vi "AlliGator Decay Fit Parameter Map Context Menu Handler.vi"(8 "Error In":errorcluster, 11 "Image Event Data":T1) -> (0 "Error Out":errorcluster, 3 "AlliGator Actions":T4[](array[typedef]))   [LabVIEW 2021, in "AlliGator Decay Fit Parameter Map.lvlib"]
doc: "Decay Fit Parameter Map contextual menu handler."
uses:
  AlliGator Decay Fit Parameter Map.lvlib
  AlliGator Q Element.ctl
  AlliGator Q Event.ctl
  Image/Image Display Event.ctl
  Image/Image Control Refnum.ctl
  <vilib>/Utility/miscctls.llb/LVPoint32TypeDef.ctl
  Image/Image Display to Clipboard Options.ctl
  AlliGator Variables List.ctl
  Files/Load-Save File Info.ctl
  Variant/Variant to Data/Variant to I32.vi
  AlliGator Action Engine.lvlib
  Image/Image.lvlib
  Files/Files.lvlib
  AlliGator Globals, Variables & Constants.lvlib
  Variant/Variant to Data/Variant to Data.lvlib
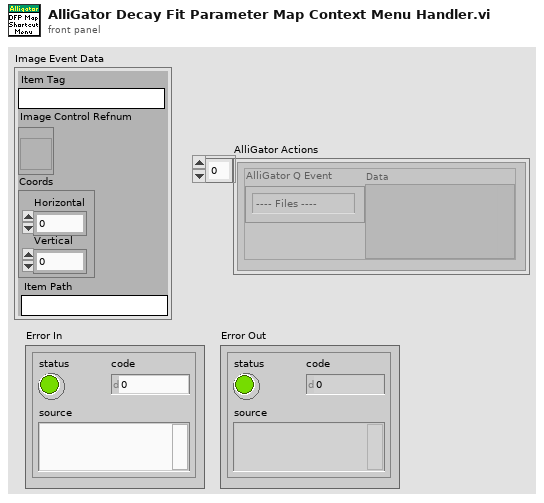
[diagram p1: front panel]
types:
  T1 = typedef "Image.lvlib/Image Display Event.ctl" = cluster{"Item Tag":string, "Image Control Refnum":T2, "Coords":T3, "Item Path":string}
  T2 = typedef "Image.lvlib/Image Control Refnum.ctl" = refnum<vi>
  T3 = typedef "LVPoint32TypeDef.ctl" = cluster{"Horizontal":i32, "Vertical":i32}
  T4 = typedef "AlliGator Action Engine.lvlib/AlliGator Q Element.ctl" = cluster{"AlliGator Q Event":T5, "Data":variant}
  T5 = typedef "AlliGator Action Engine.lvlib/AlliGator Q Event.ctl" = enum16{"---- Files ----", "Files:Set Batch Export Files To Save", "Files:Set Dataset Loading & Pre-processing Options", "Files:Check #Frames in Dataset", "Files:Increment Frame Index", "Files:Open Mask Image", "Files:Open White Light Image", "Files:Open Single Dataset", "Files:New Folder of Folders Selected", "Files:Load File (all Types)_Scriptable", "Files:Move Flattened Series to Folders Series", "Files:Select Folder", "Files:Load FLI Dataset", "Files:Load Swiss SPAD 1 Dataset", "Files:Load Swiss SPAD 2 Dataset", "Files:Load .sdt FLI Dataset", "Files:Load .ptu FLI Dataset", "Files:Load .bin FLI Dataset", "Files:Load Single Gate Image Folder", "Files:Load I/m/phi Dataset (deprecated)", "Files:Load Single Image", "Files:Subtract Background File", "Files:Export FLI Dataset", "Files:Load HDF5 FLI Dataset", "Files:Set Destination File Path", "Files:Save Mask Image", "Files:Batch Conversion", "Files:New Folder Selected", "Files:Close FLI Dataset", "Files:Close FLI Dataset Series", "Files:Close White Light Image", "Files:Close Mask Image", "---- FLI Dataset ----", "FLI Dataset:Channel Arithmetic", "FLI Dataset:Export Average Lifetime Map as ASCII", "FLI Dataset:Export User-Defined Quantity Map as ASCII", "FLI Dataset:Python Function FLI Dataset Event", "FLI Dataset:ROI Analysis", "FLI Dataset:Tilted Logistic Square Gated IRF Characteristics Map", "FLI Dataset:Logistic Square Gated IRF Characteristics Map", "FLI Dataset:Square Gated IRF Characteristics Map", "FLI Dataset:Multi-ROI Single-Pixel Phasor Analysis", "FLI Dataset:Multi-ROI Single-Pixel NLSF Analysis", "FLI Dataset:All ROIs IRF Extraction", "FLI Dataset:All ROIs Decay Fit Non-Interactive (Fast + Individual IRF)", "FLI Dataset:All ROIs Phasor Analysis", "FLI Dataset:All ROIs Decay Fit", "FLI Dataset:Fluorescence Decay Statistics", "FLI Dataset:Update Decay Statistics Graph", "FLI Dataset:Get Decay from ROI", "FLI Dataset:All ROIs Average Lifetimes", "---- FLI Dataset Series ----", "FLI Dataset Series:Sum All Datasets in Series", "FLI Dataset Series:Add Dataset to Accumulated Dataset", "FLI Dataset Series:Display Accumulated Dataset", "FLI Dataset Series:Clear Dataset Series Sum", "FLI Dataset Series:Time-Series Analysis (NLSF)", "FLI Dataset Series:Time-Series Analysis (Phasor)", "---- Image ----", "Image:Update Image Profile Plots", "Image:Image Histogram Cursor Move", "Image:Image Histogram", "Image:Image Contrast", "Image:Set Image Histogram Cursor Move Flag", "Image:Clear Image Overlay", "Image:Use ROI as Search Area", "Image:Set ROI Diameter", "Image:Save Image Data as TIFF", "Image:Save Displayed Image with Overlay", "Image:Save Image Overlay Only", "Image:Save Image as Hot Pixel Mask", "Image:Change Source Image Color Palette", "Image:Copy Image to Clipboard", "Image:Source Image ROI Selection", "Image:Delete All ROIs", "Image:Delete All Unselected ROIs", "Image:Delete ROI", "Image:Merge All ROIs", "Image:Store ROI", "Image:Source Image ROI Storage", "Image:Export ROI Description to Notebook", "Image:Save ROI", "Image:Load ROI", "Image:Paste ROI Definition", "Image:Clear ROI", "Image:Identify ROIs in Mask Image", "Image:Create Complementary ROI", "Image:Create Contour ROI", "Image:Create ROI(s) from Pixels with Peak above Min_Scriptable", "Image:Create ROI(s) from Pixels with Intensity above Min_Scriptable", "Image:Compute ROI Statistics", "Image:Delete ROI(s) based on ROI Characteristics", "Image:Create ROI Grid", "Image:ROI to Individual Pixel ROIs", "Image:Python Function Source Image Event", "Image:Show Phasor Calibration Map ROI Centers", "Image:Convert ROI to Mask Image", "Image:Mouse Move", "Image:Mouse Up", "Image:Set Source Image Mouse Move Flag", "Image:Add Scale Bar Overlay", "Image:Delete Existing ROIs Option", "---- Decay ----", "Decay:Clear IRF/Reference Plot", "Decay:Clear Local IRFs", "Decay:Add Decay to Graph", "Decay:Smoothen Plot", "Decay:Smoothen Plot Tail", "Decay:Average Selected Plots", "Decay:Extract IRF", "Decay:Optimal IRF Extraction", "Decay:Threshold IRF", "Decay:Fit to Model IRF", "Decay:Fit IRF to Square Gate", "Decay:Fit IRF to Logistic Square Gate", "Decay:Fit IRF to Tilted Logistic Square Gate", "Decay:Create Bounding Cursors Set", "Decay:Export Bounding Cursors Definition to Notebook", "Decay:Denoise Plot", "Decay:Compute Cumulative Function", "Decay:Use as Reference Decay", "Decay:Show Reference Decay/IRF", "Decay:Extrapolate Decay", "Decay:Create Head & Tail Bounding Cursors", "Decay:Store Cursor-defined Head & Tail Fractions", "Decay:Rebin Plot", "Decay:1-Normalize Decay", "Decay:[0-1]-Normalize Plot", "Decay:Straighten Decay", "Decay:Shift Decay", "Decay:Fold Decay", "Decay:Fit Decay", "Decay:Global Fit of Selected Decays", "Decay:Post Global Fit Script", "Decay:Add Global Fit Parameters to Graph", "Decay:Add Decay Parameter(s) to Plot (Graph)", "Decay:Export Decay to Phasor Graph", "Decay:Plot Decay Shifts", "Decay:Compute Average Lifetime", "Decay:Plot Convolution", "Decay:Graph Tip Strip Update", "---- Decay Statistics ----", "Decay Statistics:Tip Strip Update", "---- Intensity Time Trace ----", "Intensity Time Trace:Use File Timestamp", "Intensity Time Trace:Load Intensity Corrections File", "Intensity Time Trace:Clear Intensity Corrections File", "Intensity Time Trace:Tip Strip Update", "---- Phasor Plot ----", "Phasor Plot:Build Phasor Plot", "Phasor Plot:Change Phasor Plot Color Palette", "Phasor Plot:Adjust Phasor Plot Display Range", "Phasor Plot:Highlight Image ROI in Phasor Plot", "Phasor Plot:Save Phasor Plot Image with Overlay", "Phasor Plot:Export Complex Phasor Map", "Phasor Plot:Export Phasor Ratio Map", "Phasor Plot:Export Average Lifetime Map", "Phasor Plot:Compute Phase Lifetime Histogram", "Phasor Plot:Compute Phasor Ratio Histogram", "Phasor Plot:Compute Phase Lifetime vs Intensity Scatter Plot", "Phasor Plot:Weber 2-Component Decomposition", "Phasor Plot:Update Phasor Color Map Vertices", "Phasor Plot:Clear Phasor Overlay", "Phasor Plot:Use Segment Extremities as References", "Phasor Plot:Use UC/Segment Intersections as References", "Phasor Plot:Use UC/Principal Axis Intersections as References", "Phasor Plot:Use UC/Linear Fit Intersections as References", "Phasor Plot:Update Phasor Plot Reference", "Phasor Plot:Show Local Phasor Info in Phasor Plot", "Phasor Plot:Update Phasor Plot State", "Phasor Plot:Phasor Plot ROI Storage", "Phasor Plot:Phasor Plot ROI Selection", "Phasor Plot:Python Function Phasor Plot Event", "Phasor Plot:Overlay Phasor ROI, Ratio or Map in Source Image", "Phasor Plot:Compute Decay of Selected Phasors", "Phasor Plot:Phasor at Image Pixel", "Phasor Plot:Mouse Move", "Phasor Plot:Mouse Up", "Phasor Plot:Display Range Mouse Move", "Phasor Plot:Set Mouse Move Flag", "---- Phasor Graph ----", "Phasor Graph:Calibrated Phasor Map Series", "Phasor Graph:Whole Image Phasor Scatter Plot (Todo)", "Phasor Graph:Get Phasor Value", "Phasor Graph:Create New Phasor Plot Dialog", "Phasor Graph:Update Last Phasor Value", "Phasor Graph:Update Phasor (m, phi)", "Phasor Graph:Remove Single Phasor from Plot", "Phasor Graph:Add Single Phasor to Plot", "Phasor Graph:Remove Phasor Plot", "Phasor Graph:Remove Selected Phasor Plots", "Phasor Graph:Clear Phasor Data", "Phasor Graph:Clear Phasor Graph", "Phasor Graph:Cursor Move", "Phasor Graph:Draw Cursor Connecting Line", "Phasor Graph:Clear Cursor Connecting Line", "Phasor Graph:Find UC Intersection", "Phasor Graph:Use UC/Cursor-Defined Line Intersections", "Phasor Graph:Use Selected Plots Fitted Line/UC Intersections", "Phasor Graph:Use Selected Plots Principal Axis/UC Intersections", "Phasor Graph:Show Single Phasor", "Phasor Graph:Save Single Phasor Plot", "Phasor Graph:Save All Phasor Plots", "Phasor Graph:Load Phasor Plot(s)", "Phasor Graph:Phasor Multiplication", "Phasor Graph:Compute Average Phasor", "Phasor Graph:Compute Multiple Average Phasors (Selected Plots)", "Phasor Graph:Export Single Phasor Plot Phase Lifetimes", "Phasor Graph:Phase Lifetime Trajectory", "Phasor Graph:Phase Lifetime vs Intensity Scatter Plot (deprecated)", "Phasor Graph:Parameter 2 vs Parameter 1 Scatter Plot", "Phasor Graph:Use Cursor n Location", "Phasor Graph:Set Reference n to Current Phase Lifetime Value", "Phasor Graph:Set Reference n to Lifetime Value", "Phasor Graph:Set Cursor n Location", "Phasor Graph:Save Phasor Graph Image", "Phasor Graph:Update SEPL Plot", "Phasor Graph:Export Single Phasor Plot Data", "Phasor Graph:Export Selected Phasor Plots Data", "Phasor Graph:Python Function Phasor Graph Event", "Phasor Graph:Tip Strip Update", "---- Calibration ----", "Calibration:Set Calibration Type", "Calibration:Load/Save Phasor Calibration", "Calibration:Load/Save Phasor Calibration Series", "Calibration:Load/Save Phasor Calibration Map", "Calibration:Use as Calibration", "Calibration:Compute Optimal Calibration from Phasor References", "Calibration:Clear Phasor Calibration", "Calibration:Single Phasor Calibration Information", "Calibration:Use as Calibration Series", "Calibration:Use as Calibration Map", "Calibration:Clear Calibration Series", "Calibration:Phasor Calibration Series Information", "Calibration:Clear Calibration Map", "Calibration:Phasor Calibration Map Information", "Calibration:Apply Phasor Calibration", "Calibration:Update Single Plot Calibration", "Calibration:Update Multiple Plots Calibration", "Calibration:Clear Single Plot Calibration", "Calibration:Clear All Plots Calibrations", "Calibration:Clear Plot(s) Calibration(s)?", "Calibration:Phasor Calibration Maps (# Gates Series)", "---- Phasor Ratio ----", "Phasor Ratio:Clear Reference n", "Phasor Ratio:Toggle Selected Plot(s)  Lock to Reference 1", "Phasor Ratio:Use as Reference n", "Phasor Ratio:Send Reference n to Notebook", "Phasor Ratio:Toggle Selected Plot(s)  Lock to Reference 2", "Phasor Ratio:Compute Phasor Ratio at Mouse Location", "Phasor Ratio:Compute Phasor Plot's Average Phasor Ratio", "Phasor Ratio:Compute Time-Series Phasor Ratios", "Phasor Ratio:Fit Line to Phasor Ratio Plot", "Phasor Ratio:Save References", "Phasor Ratio:Load References", "Phasor Ratio:Update Phasor Reference 1", "Phasor Ratio:Update Phasor Reference 2", "Phasor Ratio:Move Cursor n to Reference n", "Phasor Ratio:Use as Phasor Reference 1 Lifetime", "Phasor Ratio:Use as Phasor Reference 2 Lifetime", "Phasor Ratio:Export Phasor Ratio Map as ASCII", "Phasor Ratio:Tip Strip Update", "---- Lifetime & Other Parameters Graph ----", "Lifetime:Tip Strip Update", "---- Decay Fit Parameter Map ----", "Decay Fit Parameter Map:Export ROI NLSF Data as ASCII", "Decay Fit Parameter Map:Set Decay Fit  Parameter Map Selection", "Decay Fit Parameter Map:Build Decay Fit Parameter Map", "Decay Fit Parameter Map:Change Decay Fit Parameter Map Color Palette", "Decay Fit Parameter Map:Export Decay Fit Parameter Map Data as ASCII", "Decay Fit Parameter Map:Export All Decay Fit Parameter Maps Data as ASCII", "Decay Fit Parameter Map:Send Map Data to Lifetime Graph", "Decay Fit Parameter Map:Save Decay Fit Parameter Map Image", "Decay Fit Parameter Map:Save-Load IRFs & Fit Data", "Decay Fit Parameter Map:Update Local Decay Plots", "Decay Fit Parameter Map:Python Function Decay Fit Parameters Map Event", "Decay Fit Parameter Map:Overlay Decay Fit Parameter Map in Source Image", "Decay Fit Parameter Map:Plot Map Data vs Intensity", "Decay Fit Parameter Map:Mouse Up", "Decay Fit Parameter Map:Display Range Mouse Move", "---- Generic Graph ----", "Generic Graph:Generic XY Graph Event", "Generic Graph:Python Function XY Graph Event", "Generic Graph:New Plot", "Generic Graph:Save Plot", "Generic Graph:XY Plot Histogram", "Generic Graph:Set XY Graph Plot Name", "Generic Graph:Set Last Cursor Style", "Generic Graph:Tip Strip Update", "---- GUI ----", "GUI:Start Script", "GUI:Type of Displayed Image Changed", "GUI:Gate Image Slide Changed", "GUI:Show Busy Icon", "GUI:Show Busy Icon & Abort Button", "GUI:Hide Busy Icon", "GUI:Hide Busy Icon & Abort Button", "GUI:Abort", "GUI:End Script", "GUI:Start Timing", "GUI:End Timing", "GUI:Set State Indicator", "GUI:Send Parameters JSON Strings to Clipboard", "GUI:Set Gate Step", "GUI:Idle", "GUI:Initialization", "GUI:Quit", "GUI:Increment Dataset Index", "GUI:Set Dataset Index to -1", "GUI:Time Series Slider Moved", "GUI:Time Series Slider Changed", "GUI:Toggle Playback or Loop", "GUI:Playback Script", "GUI:Set Phasor Frequency", "GUI:Open Window", "GUI:Start Test Script", "GUI:End Test Script", "DEBUG"}
  T6 = typedef "Image.lvlib/Image Display to Clipboard Options.ctl" = cluster{"Include Overlay (T)":bool, "Image Only (T)":bool}
  T7 = typedef "AlliGator Globals, Variables & Constants.lvlib/AlliGator Variables List.ctl" = enum16{"---- GUI ----", "Initialization Status", "State Indicators Refnum", "Original AlliGator Menu Items", "Current Action Loop State", "Script in progress", "Playback", "Loop Playback", "Search ROI Used", "Search ROI", "Decay Graph Max Legend Size", "Intensity Graph Max Legend Size", "Decay Statistics Graph Max Legend Size", "Phasor Graph Max Legend Size", "Phasor Ratio Graph Max Legend Size", "Lifetime Graph Max Legend Size", "---- Files ----", "Export Dataset Frames as Individual Files", "Show Batch Export Help Balloons", "Frames in Dataset", "ptu File Frame Start Indices", "Current Frame in Dataset", "Current Frame Timestamp", "------ Python Plugins ------", "Python Plugins Information", "Python Session", "Valid Python Session?", "---- Source Image ----", "Dataset Loaded", "Dataset Metadata", "Dataset Channel", "Dataset Data Description", "Background Dataset Metadata", "Background Dataset Channel", "Background Dataset Data Description", "Background File Subtraction", "Background File Path", "Background File Pile-up Correction", "Background File Pixel Well Capacity", "Background File Scaling Factor", "Source Image ROIs", "Current Source Image ROI", "Source Image ROI Event Refnum", "X_Source Image Display Range", "X_Source Image Palette Information", "Source Image Palette List", "Source Image Scale", "Current Dataset Load Settings", "Source Image:ROI Overlay Color", "---- Image Profile Window ----", "Image Profile:Overlay ROI in Source Image", "Image Profile Window Event Refnum", "Image Profile:IntensityType", "Image Profile:Intensity Average Type", "Image Profile:Intensity-weighted SDV", "Image Profile:Box Profile Type", "Image Profile Window Open", "Image Profile:Plotted Fit Parameter", "X_Type of Displayed Image", "X_Time Gate Slider", "Dataset Path", "Source Image Overlay to Erase", "Is Displayed Image Accumulated", "White Light Image Modified", "Mask Image Modified", "Macrotime Gate Separation", "------ Phasor Graph -------", "Phasor Graph:Show Line", "---- Phasor Plot ---", "Phasor Plot Parameters Changed", "FLI Dataset Modified since last Phasor Plot Calculation", "Phasor Harmonics Data", "Selected Phasor Harmonics", "Phasor Harmonic Manager Event Refnum", "Phasor Plot ROIs", "Current Phasor Plot ROI", "Phasor Plot ROI Event Refnum", "Phasor Plot Image Reference Points", "Phasor Plot Computed", "Phasor Plot Palette Information", "Phasor Plot Palette List", "Phasor Ratio Palette Information", "Phasor Ratio Palette List", "Phasor Image Scale", "Phasor Plot Image Overlay to Erase", "Phasor Plot Image Elements to Update", "Current Phasor Plot Calculation Parameters", "Current Phasor Calibration Options", "Reset Cumulated Phasor Plot", "Phasor Ratio Reference 1", "Phasor Ratio Lifetime Reference 1", "Phasor Ratio Reference 1 Frequency", "Phasor Ratio Reference 2", "Phasor Ratio Lifetime Reference 2", "Phasor Ratio Reference 2 Frequency", "---- Decay Analysis ----", "Number of Selected Decays to Fit", "LS Fit Results", "LAR Fit Results", "BS Fit Results", "Last Decay Max - Min", "Best Fit Parameters", "Best Fit Parameter Names", "Actual Size X", "Actual Size Y", "Binning X", "Binning Y", "Actual # Gates", "Dataset Number", "Gates to...", "Gates Skipped", "Gates to keep", "Gate Step", "Gate Separation", "Reversed Gates", "Pile-up Correction", "Pixel Well Capacity", "Background Subtracted", "Background Subtraction Method", "Background Definition Range", "Background File (deprecated)", "Number of Dataset Accumulated", "Array of Accumulated Dataset Paths", "Do Averaged Datasets", "Destination File Path", "Process Plot Target", "Use 1/D as Phasor Frequency", "---- Decay Fit Parameter Map -----", "Decay Fit Parameter Map Palette Information", "Decay Fit Parameter Map Palette List", "Local Decay Graph Window Event Refnum", "------- Local Decay Window ---------", "Use normalized IRF for convolution", "----- Miscellaneous ----", "Skippable Dialog Windows Status"}
  T8 = typedef "Files.lvlib/Load-Save File Info.ctl" = cluster{"Load/Save":bool, "File Path":path}
  T9 = cluster{"Image Control Refnum":T2, "Image to Clipboard Options":T6}
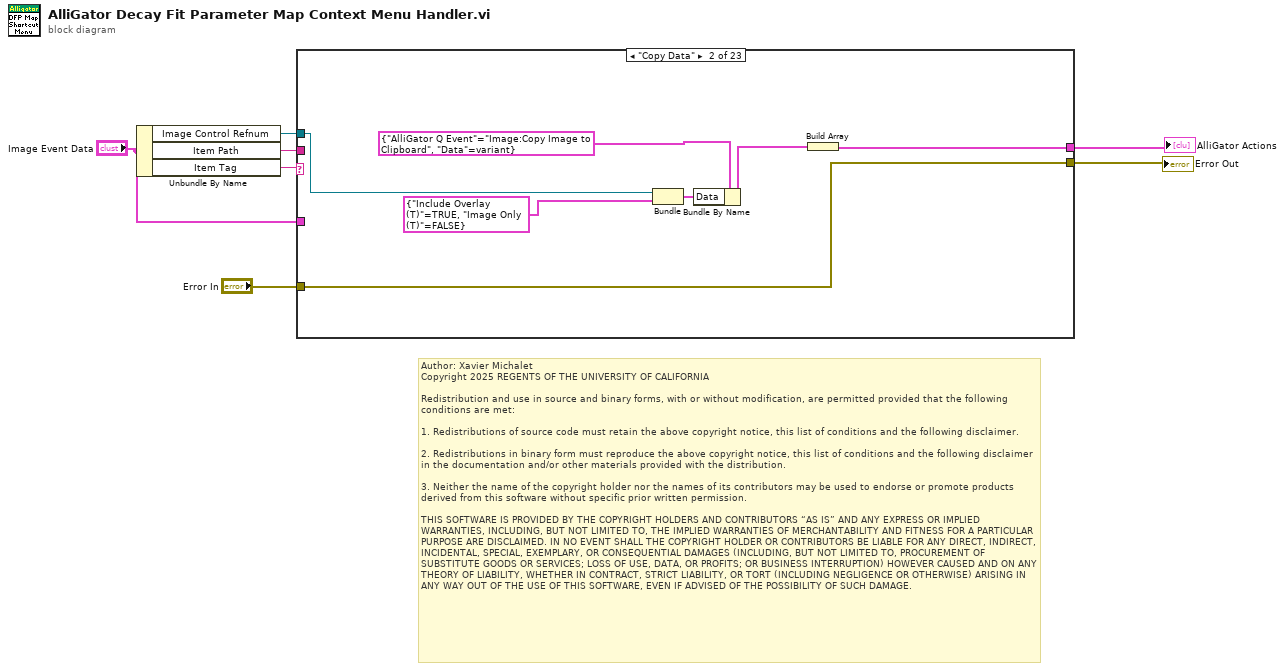
[diagram p0: block diagram]
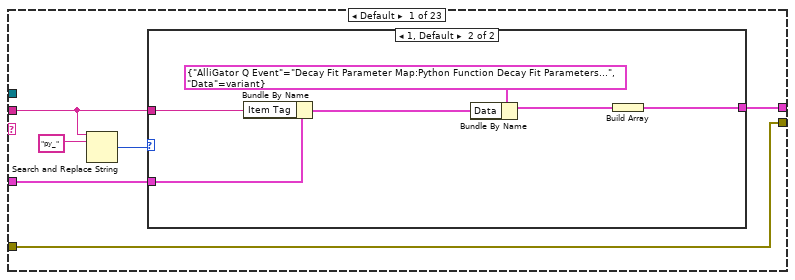
[diagram p2: hidden frame]
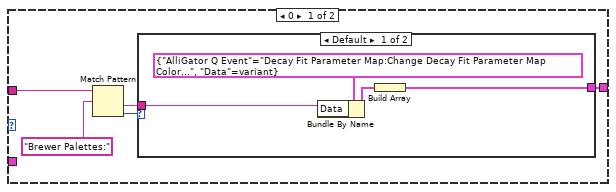
[diagram p3: hidden frame]
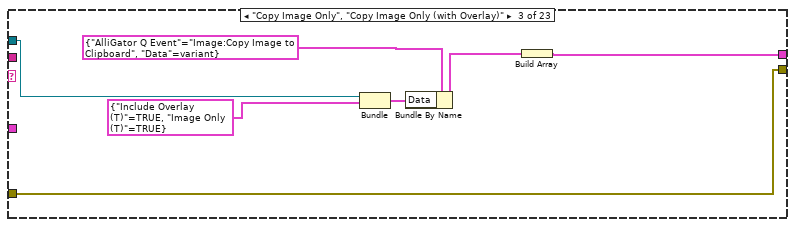
[diagram p5: hidden frame]
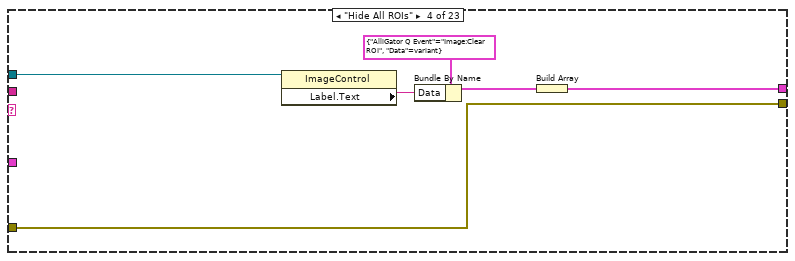
[diagram p6: hidden frame]
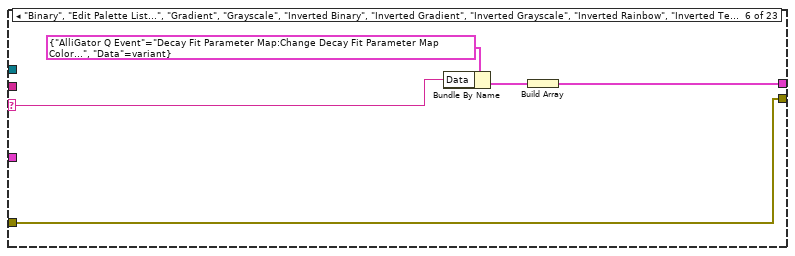
[diagram p8: hidden frame]
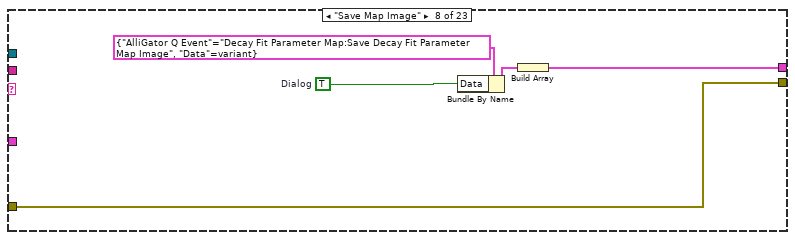
[diagram p10: hidden frame]
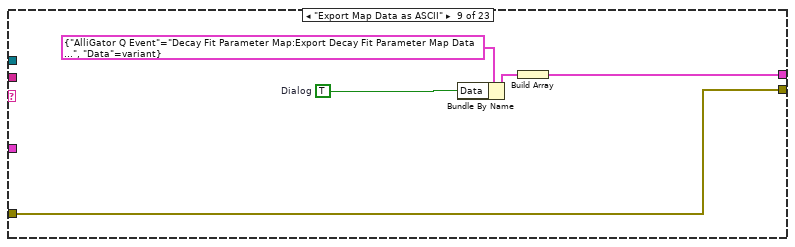
[diagram p11: hidden frame]
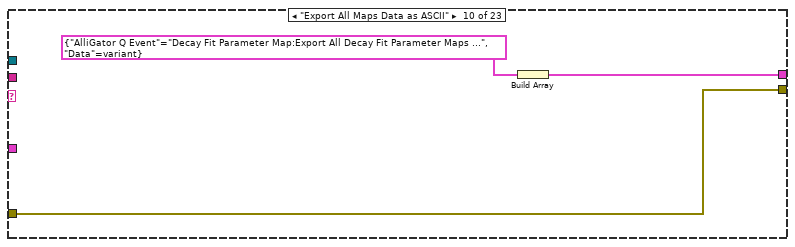
[diagram p12: hidden frame]
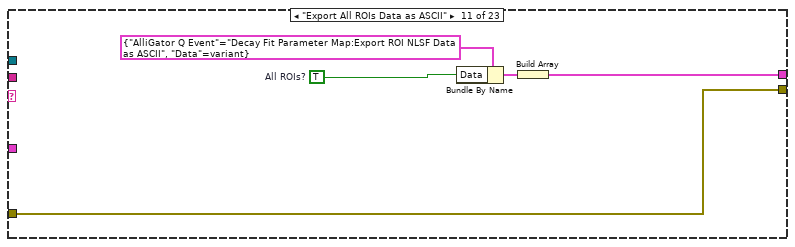
[diagram p13: hidden frame]
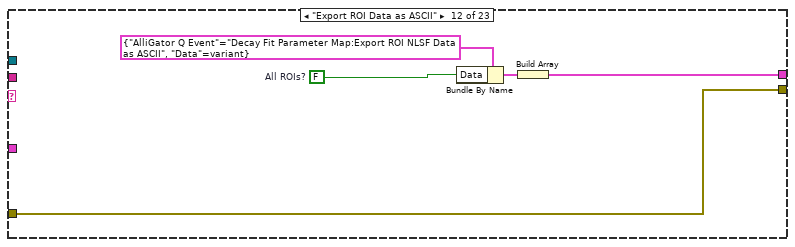
[diagram p14: hidden frame]
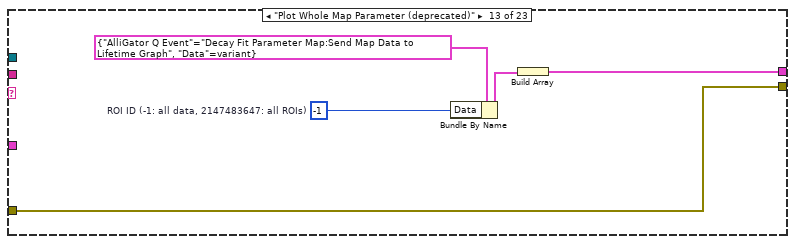
[diagram p15: hidden frame]
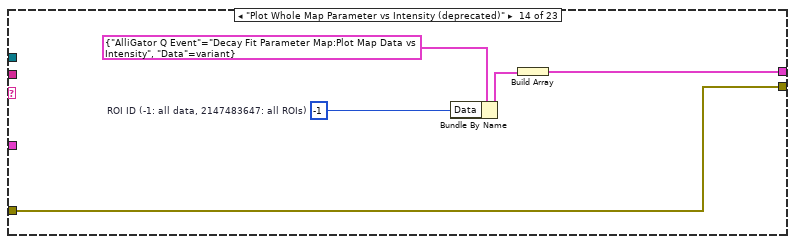
[diagram p16: hidden frame]
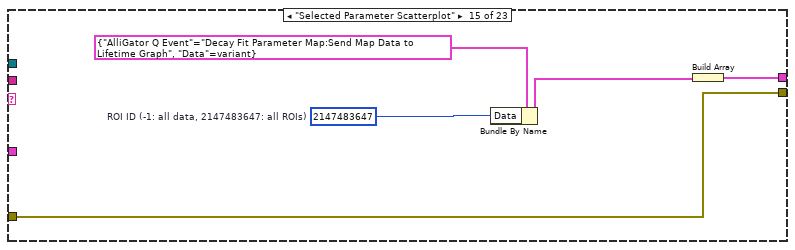
[diagram p17: hidden frame]
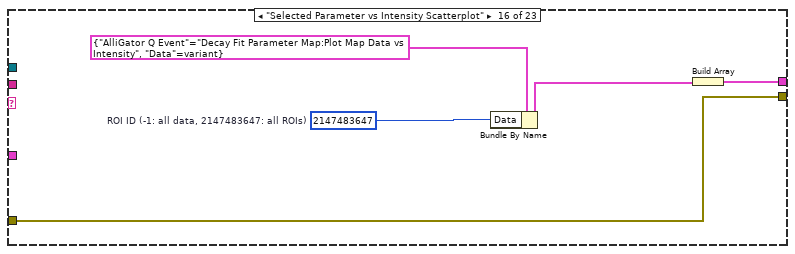
[diagram p18: hidden frame]
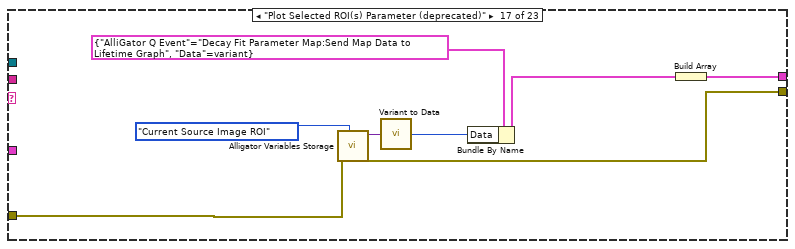
[diagram p19: hidden frame]
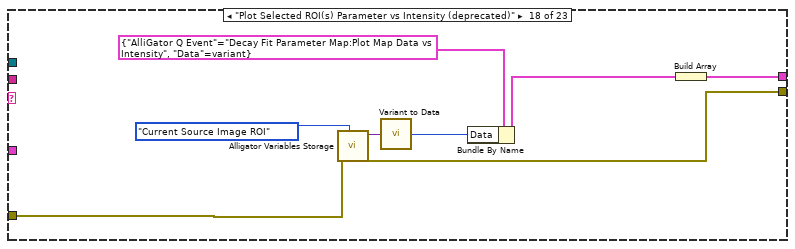
[diagram p20: hidden frame]
diagram:
  # "Author: Xavier Michalet\nCopyright 2025 REGENTS OF THE UNIVERSITY OF CALIFORNIA\n\nRedistribution and use in source and binary forms, with or without modification, are permitted provided that the following conditions are met:\n\n1. Redistributions of source code must retain the above copyright notice, this list of conditions and the following disclaimer.\n\n2. Redistributions in binary form must reproduce the above copyright notice, this list of conditions and the following disclaimer in the documentation and/or other materials provided with the distribution.\n\n3. Neither the name of the copyright holder nor the names of its contributors may be used to endorse or promote products derived from this software without specific prior written permission.\n\nTHIS SOFTWARE IS PROVIDED BY THE COPYRIGHT HOLDERS AND CONTRIBUTORS “AS IS” AND ANY EXPRESS OR IMPLIED WARRANTIES, INCLUDING, BUT NOT LIMITED TO, THE IMPLIED WARRANTIES OF MERCHANTABILITY AND FITNESS FOR A PARTICULAR PURPOSE ARE DISCLAIMED. IN NO EVENT SHALL THE COPYRIGHT HOLDER OR CONTRIBUTORS BE LIABLE FOR ANY DIRECT, INDIRECT, INCIDENTAL, SPECIAL, EXEMPLARY, OR CONSEQUENTIAL DAMAGES (INCLUDING, BUT NOT LIMITED TO, PROCUREMENT OF SUBSTITUTE GOODS OR SERVICES; LOSS OF USE, DATA, OR PROFITS; OR BUSINESS INTERRUPTION) HOWEVER CAUSED AND ON ANY THEORY OF LIABILITY, WHETHER IN CONTRACT, STRICT LIABILITY, OR TORT (INCLUDING NEGLIGENCE OR OTHERWISE) ARISING IN ANY WAY OUT OF THE USE OF THIS SOFTWARE, EVEN IF ADVISED OF THE POSSIBILITY OF SUCH DAMAGE."
  n1 = Unbundle By Name("Image Event Data") -> ("Image Control Refnum"=w4:T2, "Item Path"=w3:string, "Item Tag"=w2:string)
  n2 = case shown="\"Copy Data\"" w2 {
    selector: w2 -> [_ _ _ _ _ w52 _ _ _ _ _ _ _ _ _ _ _ _ _ _ _ _ _]
    tunnel: w4 -> [_ w31 w38 w43 _ _ _ _ _ _ _ _ _ _ _ _ _ _ _ _ _ w132 w134]
    tunnel: w3 -> [w8 _ _ _ _ _ _ _ _ _ _ _ _ _ _ _ _ _ _ _ _ _ _]
    tunnel: [w13 w30 w37 w44 _ w51 _ w57 w62 w67 w72 w77 w82 w87 w92 w97 w106 w114 w120 w127 _ _ _] -> w7
    tunnel: "Error In" -> [w12 w29 w36 w48 w49 w50 w55 w60 w65 w68 w73 w78 w83 w88 w93 w98 w102 w110 w121 w128 w129 w130 w133]
    tunnel: [w12 w29 w36 w48 w49 w50 w55 w60 w65 w68 w73 w78 w83 w88 w93 w98 w101 w109 w121 w128 w129 w130 w133] -> w5
    tunnel: "Image Event Data" -> [w9 _ _ _ _ _ _ _ _ _ _ _ _ _ _ _ _ _ _ _ _ _ _]
    frame Default {
      n3 = Search and Replace String(input string=w8, search string="py_") -> (number of replacements=w10:i32)  [unwired: 6 in, 3 out]
      n4 = case shown="1, Default" w10 {
        tunnel: [w15 w23] -> w13
        tunnel: w8 -> [w14 w26]
        tunnel: w9 -> [_ w24]
        frame 0 {
          n5 = Match Pattern(string=w14, regular expression="Brewer Palettes:") -> (after substring=w16:string, offset past match=w17:i32)  [unwired: 1 in, 2 out]
          n6 = case shown="Default" w17 {
            tunnel: w16 -> [w20 _]
            tunnel: [w19 _] -> w15
            frame Default {
              n7 = Bundle By Name(cluster=T4 {"AlliGator Q Event"=enum."Decay Fit Parameter Map:Change Decay Fit Parameter Map Color Palette", "Data"=variant} ("element"), "Data"=w20) -> (w21:T4)
              n8 = Build Array(w21) -> (w19:T4[])
            }
            frame -1 {
            }
          }
        }
        frame 1, Default {
          n9 = Bundle By Name(cluster=w24, "Item Tag"=w26) -> (w27:T1)
          n10 = Bundle By Name(cluster=T4 {"AlliGator Q Event"=enum."Decay Fit Parameter Map:Python Function Decay Fit Parameters Map Event", "Data"=variant}, "Data"=w27) -> (w25:T4)
          n11 = Build Array(w25) -> (w23:T4[])
        }
      }
    }
    frame "Copy Data" {
      n12 = Bundle("Image Control Refnum"=w31, "Image to Clipboard Options"=T6 {"Include Overlay (T)"=TRUE, "Image Only (T)"=FALSE}) -> (w32:T9)  [unwired: 1 in]
      n13 = Bundle By Name(cluster=T4 {"AlliGator Q Event"=enum."Image:Copy Image to Clipboard", "Data"=variant} ("element"), "Data"=w32) -> (w34:T4)
      n14 = Build Array(w34) -> (w30:T4[])
    }
    frame "Copy Image Only", "Copy Image Only (with Overlay)" {
      n15 = Bundle("Image Control Refnum"=w38, "Image to Clipboard Options"=T6 {"Include Overlay (T)"=TRUE, "Image Only (T)"=TRUE}) -> (w39:T9)  [unwired: 1 in]
      n16 = Bundle By Name(cluster=T4 {"AlliGator Q Event"=enum."Image:Copy Image to Clipboard", "Data"=variant} ("element"), "Data"=w39) -> (w41:T4)
      n17 = Build Array(w41) -> (w37:T4[])
    }
    frame "Hide All ROIs" {
      n18 = property class="ImageControl"(reference=w43) -> ("Label.Text"=w45:string)  [unwired: 1 in, 2 out]
      n19 = Bundle By Name(cluster=T4 {"AlliGator Q Event"=enum."Image:Clear ROI", "Data"=variant} ("element"), "Data"=w45) -> (w46:T4)
      n20 = Build Array(w46) -> (w44:T4[])
    }
    frame "---------Palette----------" {
    }
    frame "Binary", "Edit Palette List...", "Gradient", "Grayscale", "Inverted Binary", "Inverted Gradient", "Inverted Grayscale", "Inverted Rainbow", "Inverted Temperature", "Rainbow", "Select New Palette...", "Temperature" {
      n21 = Bundle By Name(cluster=T4 {"AlliGator Q Event"=enum."Decay Fit Parameter Map:Change Decay Fit Parameter Map Color Palette", "Data"=variant} ("element"), "Data"=w52) -> (w53:T4)
      n22 = Build Array(w53) -> (w51:T4[])
    }
    frame "--------- Others  ---------" {
    }
    frame "Save Map Image" {
      w56 = TRUE  # Dialog
      n23 = Bundle By Name(cluster=T4 {"AlliGator Q Event"=enum."Decay Fit Parameter Map:Save Decay Fit Parameter Map Image", "Data"=variant} ("Time-Gated Phasor Q Element"), "Data"=w56) -> (w58:T4)
      n24 = Build Array(w58) -> (w57:T4[])
    }
    frame "Export Map Data as ASCII" {
      w61 = TRUE  # Dialog
      n25 = Bundle By Name(cluster=T4 {"AlliGator Q Event"=enum."Decay Fit Parameter Map:Export Decay Fit Parameter Map Data as ASCII", "Data"=variant} ("Time-Gated Phasor Q Element"), "Data"=w61) -> (w63:T4)
      n26 = Build Array(w63) -> (w62:T4[])
    }
    frame "Export All Maps Data as ASCII" {
      n27 = Build Array(T4 {"AlliGator Q Event"=enum."Decay Fit Parameter Map:Export All Decay Fit Parameter Maps Data as ASCII", "Data"=variant} ("Time-Gated Phasor Q Element")) -> (w67:T4[])
    }
    frame "Export All ROIs Data as ASCII" {
      w69 = TRUE  # All ROIs?
      n28 = Bundle By Name(cluster=T4 {"AlliGator Q Event"=enum."Decay Fit Parameter Map:Export ROI NLSF Data as ASCII", "Data"=variant} ("Time-Gated Phasor Q Element"), "Data"=w69) -> (w70:T4)
      n29 = Build Array(w70) -> (w72:T4[])
    }
    frame "Export ROI Data as ASCII" {
      w74 = FALSE  # All ROIs?
      n30 = Bundle By Name(cluster=T4 {"AlliGator Q Event"=enum."Decay Fit Parameter Map:Export ROI NLSF Data as ASCII", "Data"=variant} ("Time-Gated Phasor Q Element"), "Data"=w74) -> (w75:T4)
      n31 = Build Array(w75) -> (w77:T4[])
    }
    frame "Plot Whole Map Parameter (deprecated)" {
      w79 = -1  # ROI ID (-1: all data, 2147483647: all ROIs)
      n32 = Bundle By Name(cluster=T4 {"AlliGator Q Event"=enum."Decay Fit Parameter Map:Send Map Data to Lifetime Graph", "Data"=variant} ("Time-Gated Phasor Q Element"), "Data"=w79) -> (w80:T4)
      n33 = Build Array(w80) -> (w82:T4[])
    }
    frame "Plot Whole Map Parameter vs Intensity (deprecated)" {
      w84 = -1  # ROI ID (-1: all data, 2147483647: all ROIs)
      n34 = Bundle By Name(cluster=T4 {"AlliGator Q Event"=enum."Decay Fit Parameter Map:Plot Map Data vs Intensity", "Data"=variant} ("Time-Gated Phasor Q Element"), "Data"=w84) -> (w85:T4)
      n35 = Build Array(w85) -> (w87:T4[])
    }
    frame "Selected Parameter Scatterplot" {
      w89 = 2147483647  # ROI ID (-1: all data, 2147483647: all ROIs)
      n36 = Bundle By Name(cluster=T4 {"AlliGator Q Event"=enum."Decay Fit Parameter Map:Send Map Data to Lifetime Graph", "Data"=variant} ("Time-Gated Phasor Q Element"), "Data"=w89) -> (w90:T4)
      n37 = Build Array(w90) -> (w92:T4[])
    }
    frame "Selected Parameter vs Intensity Scatterplot" {
      w94 = 2147483647  # ROI ID (-1: all data, 2147483647: all ROIs)
      n38 = Bundle By Name(cluster=T4 {"AlliGator Q Event"=enum."Decay Fit Parameter Map:Plot Map Data vs Intensity", "Data"=variant} ("Time-Gated Phasor Q Element"), "Data"=w94) -> (w95:T4)
      n39 = Build Array(w95) -> (w97:T4[])
    }
    frame "Plot Selected ROI(s) Parameter (deprecated)" {
      n40 = call "Alligator Variables Storage.vi"("AlliGator Variable"=AlliGator_Variables_List."Current Source Image ROI" ("Alligator Variable"), "Error In"=w102) -> ("Error Out"=w101:errorcluster, "Data out"=w103:variant)  [unwired: 7 in, 1 out]
      n41 = call-poly "Variant to Data.vi"("Variant"=w103) -> ("Value"=w99:i32)  [unwired: 8 in]
      n42 = Bundle By Name(cluster=T4 {"AlliGator Q Event"=enum."Decay Fit Parameter Map:Send Map Data to Lifetime Graph", "Data"=variant} ("Time-Gated Phasor Q Element"), "Data"=w99) -> (w104:T4)
      n43 = Build Array(w104) -> (w106:T4[])
    }
    frame "Plot Selected ROI(s) Parameter vs Intensity (deprecated)" {
      n44 = call "Alligator Variables Storage.vi"("AlliGator Variable"=AlliGator_Variables_List."Current Source Image ROI" ("Alligator Variable"), "Error In"=w110) -> ("Error Out"=w109:errorcluster, "Data out"=w111:variant)  [unwired: 7 in, 1 out]
      n45 = call-poly "Variant to Data.vi"("Variant"=w111) -> ("Value"=w107:i32)  [unwired: 8 in]
      n46 = Bundle By Name(cluster=T4 {"AlliGator Q Event"=enum."Decay Fit Parameter Map:Plot Map Data vs Intensity", "Data"=variant} ("Time-Gated Phasor Q Element"), "Data"=w107) -> (w112:T4)
      n47 = Build Array(w112) -> (w114:T4[])
    }
    frame "Save IRFs & Fit Data" {
      n48 = Bundle By Name(cluster=T8 {"Load/Save"=FALSE, "File Path"=path ""} ("Calibration File Information"), "Load/Save"=TRUE) -> (w115:T8)
      n49 = Bundle By Name(cluster=T4 {"AlliGator Q Event"=enum."Decay Fit Parameter Map:Save-Load IRFs & Fit Data", "Data"=variant} ("Time-Gated Phasor Q Element"), "Data"=w115) -> (w118:T4)
      n50 = Build Array(w118) -> (w120:T4[])
    }
    frame "Load IRFs & Fit Data" {
      n51 = Bundle By Name(cluster=T8 {"Load/Save"=FALSE, "File Path"=path ""} ("Calibration File Information"), "Load/Save"=FALSE) -> (w124:T8)
      n52 = Bundle By Name(cluster=T4 {"AlliGator Q Event"=enum."Decay Fit Parameter Map:Save-Load IRFs & Fit Data", "Data"=variant} ("Time-Gated Phasor Q Element"), "Data"=w124) -> (w125:T4)
      n53 = Build Array(w125) -> (w127:T4[])
    }
    frame "--------------" {
    }
    frame "Zoom to Fit" {
      n54 = call "Image Display Zoom to Fit.vi"("Keep Aspect Ratio (T)"=FALSE, "Display Image Control Refnum"=w132) -> ()  [unwired: 9 in, 1 out]
    }
    frame "Zoom to Fit (Keep Aspect Ratio)" {
      n55 = call "Image Display Zoom to Fit.vi"("Display Image Control Refnum"=w134) -> ()  [unwired: 10 in, 1 out]
    }
  }
  "Error Out" <- w5
  "AlliGator Actions" <- w7
